vi "Working Point 3 Selection Dialog.vi"(7 "DisplayFilter":u8(ring)=7 items=["K_CHAN_R", "K_CHAN_W", "K_CHAN_RW", "K_CHAN_VOLT", "K_CHAN_FAULT", "K_ALL", "K_CUSTOM", "K_CHAN_R_VIS", "K_CHAN_W_VIS", "K_CHAN_RW_VIS", "K_CHAN_VOLT_VIS", "K_CHAN_FAULT_VIS"], 8 "error in (no error)":errorcluster, 9 "NIVS.System Definition Root":refnum<k24>, 10 "NodePaths":string[](array[string])) -> (0 "error out":errorcluster, 2 "Selected NodePaths":string[](array[string]))   [LabVIEW 2011]
doc: "Use this template to create a dialog box with event handling."
uses:
  NationalInstruments.VeriStand.SystemStorageUI
  NationalInstruments.VeriStand.SystemStorage
  <vilib>/NI Veristand/UI Controls/Single Node Browser/Net Event Data.ctl
  <vilib>/NI Veristand/UI Controls/Single Node Browser/Net Event.ctl
  <vilib>/NI Veristand/UI Controls/Single Node Browser/NI_VS UI Single Node Browser.lvlib
panel:
  in  "Z Value":refnum<k24>(container)
  in  "Y Index":refnum<k24>(container)
  in  "Cancel":bool
  in  "Ok":bool
  in  "X Index":refnum<k24>(container)
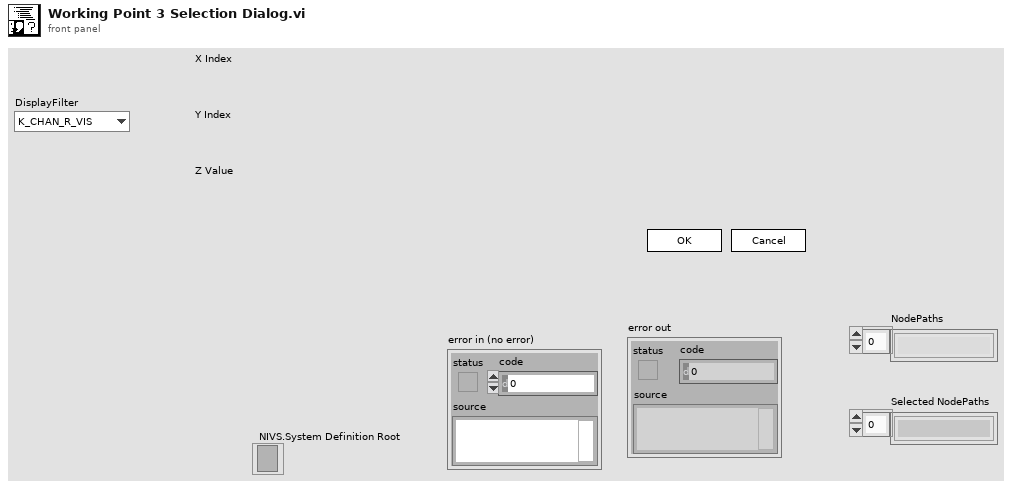
[diagram p1: front panel]
types:
  T1 = typedef "NI_VS UI Single Node Browser.lvlib/Callback Type.ctl" = cluster{"Net Callbacks":refnum<k27>[], "Event":refnum<user-event>}
  T2 = typedef "NI_VS UI Single Node Browser.lvlib/Node Ref.ctl" = refnum<k24>
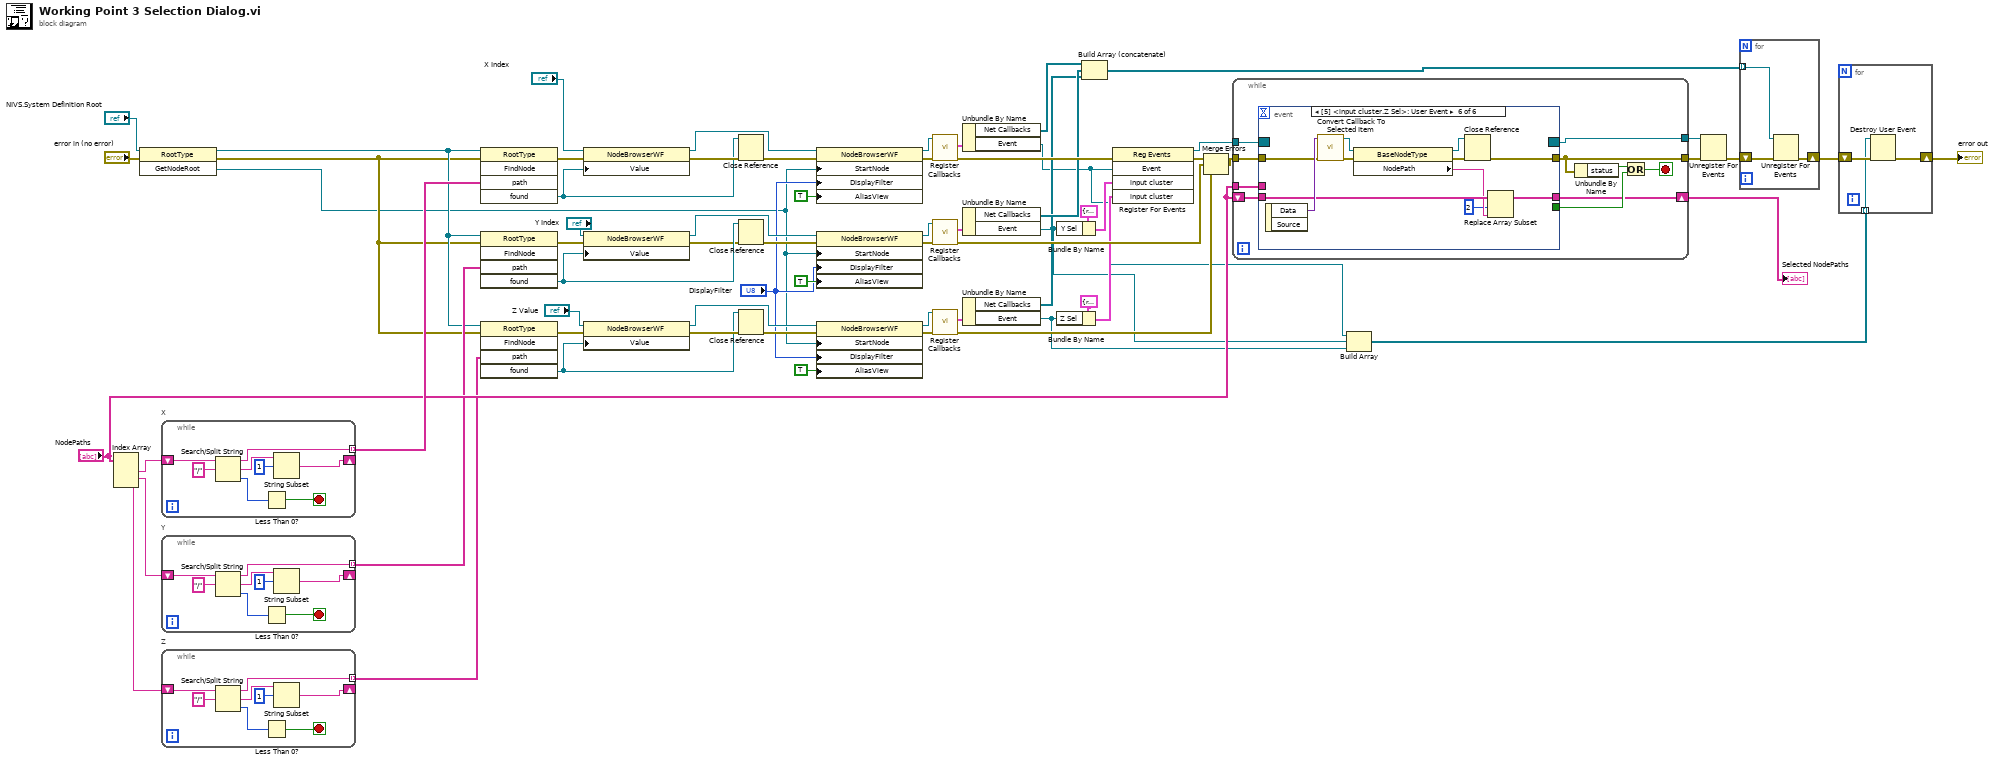
[diagram p0: block diagram]
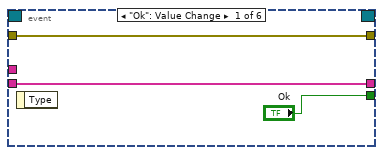
[diagram p2: hidden frame]
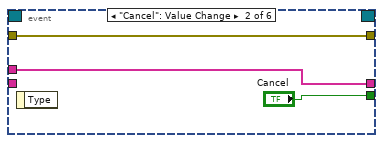
[diagram p3: hidden frame]
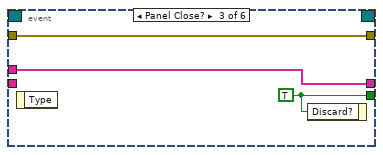
[diagram p4: hidden frame]
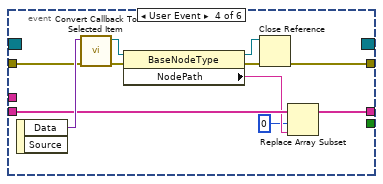
[diagram p5: hidden frame]
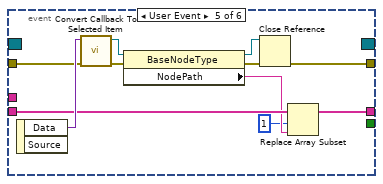
[diagram p6: hidden frame]
diagram:
  n1 = Index Array(array="NodePaths") -> (element #1=w47:string, element #2=w46:string, element #3=w26:string)  [unwired: 3 in]
  n2 = invoke class="RootType" method="GetNodeRoot"(reference="NIVS.System Definition Root", error in="error in (no error)") -> (reference out=w14:refnum<k24>, error out=w13:errorcluster, "GetNodeRoot"=w1:refnum<k24>)  [unwired: 1 in]
  n3 = while "X" {
    tunnel: [w71] -> w53 mode=indexing
    shift-right: [w69] -> _
    shift-left: w47 -> [w75]
    stop <- w72 stop-if-true
    n4 = Search/Split String(string=w75, search string/char (-)="/") -> (substring before match=w71:string, match + rest of string=w70:string, offset of match=w73:i32)  [unwired: 1 in]
    n5 = Less Than 0?(x=w73) -> (x < 0?=w72:bool)
    n6 = String Subset(string=w70, offset (0)=1) -> (substring=w69:string)  [unwired: 1 in]
  }
  n7 = while "Y" {
    tunnel: [w79] -> w34 mode=indexing
    shift-right: [w77] -> _
    shift-left: w46 -> [w83]
    stop <- w80 stop-if-true
    n8 = Search/Split String(string=w83, search string/char (-)="/") -> (substring before match=w79:string, match + rest of string=w78:string, offset of match=w81:i32)  [unwired: 1 in]
    n9 = Less Than 0?(x=w81) -> (x < 0?=w80:bool)
    n10 = String Subset(string=w78, offset (0)=1) -> (substring=w77:string)  [unwired: 1 in]
  }
  n11 = while "Z" {
    tunnel: [w87] -> w12 mode=indexing
    shift-right: [w85] -> _
    shift-left: w26 -> [w91]
    stop <- w88 stop-if-true
    n12 = Search/Split String(string=w91, search string/char (-)="/") -> (substring before match=w87:string, match + rest of string=w86:string, offset of match=w89:i32)  [unwired: 1 in]
    n13 = Less Than 0?(x=w89) -> (x < 0?=w88:bool)
    n14 = String Subset(string=w86, offset (0)=1) -> (substring=w85:string)  [unwired: 1 in]
  }
  n15 = invoke class="RootType" method="FindNode"(reference=w14, error in=w13, "path"=w53) -> (error out=w59:errorcluster, "found"=w54:refnum<k24>)  [unwired: 2 in, 3 out]
  n16 = invoke class="RootType" method="FindNode"(reference=w14, error in=w13, "path"=w34) -> (error out=w40:errorcluster, "found"=w43:refnum<k24>)  [unwired: 2 in, 3 out]
  n17 = invoke class="RootType" method="FindNode"(reference=w14, error in=w13, "path"=w12) -> (error out=w21:errorcluster, "found"=w18:refnum<k24>)  [unwired: 2 in, 3 out]
  n18 = property class="NodeBrowserWF"(reference="X Index", error in=w59, "Value"=w54) -> (reference out=w48:refnum<k24>, error out=w56:errorcluster)
  n19 = property class="NodeBrowserWF"(reference="Y Index", error in=w40, "Value"=w43) -> (reference out=w44:refnum<k24>, error out=w41:errorcluster)
  n20 = property class="NodeBrowserWF"(reference="Z Value", error in=w21, "Value"=w18) -> (reference out=w17:refnum<k24>, error out=w20:errorcluster)
  n21 = Close Reference(reference=w54, error in (no error)=w56) -> (error out=w55:errorcluster)
  n22 = Close Reference(reference=w43, error in (no error)=w41) -> (error out=w42:errorcluster)
  n23 = Close Reference(reference=w18, error in (no error)=w20) -> (error out=w19:errorcluster)
  n24 = property class="NodeBrowserWF"(reference=w48, error in=w55, "StartNode"=w1, "DisplayFilter"="DisplayFilter", "AliasView"=TRUE) -> (reference out=w61:refnum<k24>, error out=w62:errorcluster)
  n25 = property class="NodeBrowserWF"(reference=w44, error in=w42, "StartNode"=w1, "DisplayFilter"="DisplayFilter", "AliasView"=TRUE) -> (reference out=w38:refnum<k24>, error out=w37:errorcluster)
  n26 = property class="NodeBrowserWF"(reference=w17, error in=w19, "StartNode"=w1, "DisplayFilter"="DisplayFilter", "AliasView"=TRUE) -> (reference out=w23:refnum<k24>, error out=w24:errorcluster)
  n27 = call <vilib>:"Register Callbacks.vi"("error in (no error)"=w62, "Single Node Browser"=w61) -> ("error out"=w67:errorcluster, "Callbacks"=w63:T1)  [unwired: 7 in, 1 out]
  n28 = call <vilib>:"Register Callbacks.vi"("error in (no error)"=w37, "Single Node Browser"=w38) -> ("error out"=w30:errorcluster, "Callbacks"=w36:T1)  [unwired: 7 in, 1 out]
  n29 = call <vilib>:"Register Callbacks.vi"("error in (no error)"=w24, "Single Node Browser"=w23) -> ("error out"=w8:errorcluster, "Callbacks"=w25:T1)  [unwired: 7 in, 1 out]
  n30 = Unbundle By Name(w63) -> ("Net Callbacks"=w49:refnum<k27>[], "Event"=w5:refnum<user-event>)
  n31 = Unbundle By Name(w36) -> ("Net Callbacks"=w32:refnum<k27>[], "Event"=w4:refnum<user-event>)
  n32 = Unbundle By Name(w25) -> ("Net Callbacks"=w9:refnum<k27>[], "Event"=w3:refnum<user-event>)
  n33 = Bundle By Name(cluster=cluster{"Y Sel":refnum<user-event>} {"Y Sel"=refnum} ("input cluster"), "Y Sel"=w4) -> (w27:cluster{"Y Sel":refnum<user-event>})
  n34 = Bundle By Name(cluster=cluster{"Z Sel":refnum<user-event>} {"Z Sel"=refnum} ("input cluster"), "Z Sel"=w3) -> (w10:cluster{"Z Sel":refnum<user-event>})
  n35 = Build Array (concatenate)(w49, w32, w9) -> (w33:refnum<k27>[])
  n36 = register-events(error in=w67, w5, w27, w10) -> (reference out=w66:refnum<event-registration>, error out=w57:errorcluster)  [unwired: 1 in]
  n37 = Merge Errors(w57, w30, w8) -> (w31:errorcluster)
  n38 = while {
    tunnel: [w99] -> w52
    tunnel: w31 -> [w100]
    tunnel: w66 -> [w96]
    shift-right: [w95] -> w29
    shift-left: "NodePaths" -> [w94]
    tunnel: "NodePaths" -> [w93]
    tunnel: [w92] -> w51
    stop <- w98 stop-if-true
    n39 = event shown="[5] <input cluster.Z Sel>: User Event" {
      selector: w96 -> [_ _ _ _ _ _]
      dyn-events: [_ _ _ _ _ _] -> w92
      timeout: _ -> [_ _ _ _ _ _]
      tunnel: ["Ok" "Cancel" w110 _ _ _] -> w101
      tunnel: [w104 w106 w109 w119 w130 w141] -> w99
      tunnel: w100 -> [w104 w106 w109 w120 w131 w142]
      tunnel: [w102 w105 w108 w113 w124 w135] -> w95
      tunnel: w94 -> [w102 _ _ w114 w125 w136]
      tunnel: w93 -> [_ w105 w108 _ _ _]
      event "Ok": Value Change {
        n40 = event-data() -> ()  [unwired: 1 in, 1 out]
      }
      event "Cancel": Value Change {
        n41 = event-data() -> ()  [unwired: 1 in, 1 out]
      }
      event Panel Close? {
        w110 = TRUE ("Cancel")
        n42 = event-data() -> ()  [unwired: 1 in, 1 out]
        n43 = event-data("Discard?"=w110) -> ()  [unwired: 1 in, 1 out]
      }
      event User Event {
        n44 = event-data() -> ("Data"=w121:variant)  [unwired: 1 in, 1 out]
        n45 = call <vilib>:"Convert Callback To Selected Item.vi"("error in"=w120, "Data"=w121) -> ("error out"=w115:errorcluster, "Selected Item"=w118:T2)  [unwired: 8 in]
        n46 = property class="BaseNodeType"(reference=w118, error in=w115) -> (reference out=w117:T2, error out=w116:errorcluster, "NodePath"=w112:string)
        n47 = Close Reference(reference=w117, error in (no error)=w116) -> (error out=w119:errorcluster)
        n48 = Replace Array Subset(array=w114, new element=w112, index=0) -> (w113:string[])
      }
      event User Event {
        n49 = event-data() -> ("Data"=w132:variant)  [unwired: 1 in, 1 out]
        n50 = call <vilib>:"Convert Callback To Selected Item.vi"("error in"=w131, "Data"=w132) -> ("error out"=w126:errorcluster, "Selected Item"=w129:T2)  [unwired: 8 in]
        n51 = property class="BaseNodeType"(reference=w129, error in=w126) -> (reference out=w128:T2, error out=w127:errorcluster, "NodePath"=w123:string)
        n52 = Close Reference(reference=w128, error in (no error)=w127) -> (error out=w130:errorcluster)
        n53 = Replace Array Subset(array=w125, new element=w123, index=1) -> (w124:string[])
      }
      event User Event {
        n54 = event-data() -> ("Data"=w143:variant)  [unwired: 1 in, 1 out]
        n55 = call <vilib>:"Convert Callback To Selected Item.vi"("error in"=w142, "Data"=w143) -> ("error out"=w137:errorcluster, "Selected Item"=w140:T2)  [unwired: 8 in]
        n56 = property class="BaseNodeType"(reference=w140, error in=w137) -> (reference out=w139:T2, error out=w138:errorcluster, "NodePath"=w134:string)
        n57 = Close Reference(reference=w139, error in (no error)=w138) -> (error out=w141:errorcluster)
        n58 = Replace Array Subset(array=w136, new element=w134, index=2) -> (w135:string[])
      }
    }
    n59 = Unbundle By Name(w99) -> ("status"=w97:bool)
    n60 = Or(x=w97, y=w101) -> (x .or. y?=w98:bool)
  }
  "Selected NodePaths" <- w29
  n61 = Build Array(w5, w4, w3) -> (w2:refnum<user-event>[])
  n62 = Unregister For Events(event registration refnum=w51, error in=w52) -> (error out=w50:errorcluster)
  n63 = for {
    tunnel: w33 -> [w145] mode=indexing
    shift-right: [w144] -> w7
    shift-left: w50 -> [w146]
    n64 = Unregister For Events(event registration refnum=w145, error in=w146) -> (error out=w144:errorcluster)
  }
  n65 = for {
    shift-right: [w148] -> w6
    shift-left: w7 -> [w149]
    tunnel: w2 -> [w147] mode=indexing
    n66 = Destroy User Event(user event=w147, error in=w149) -> (error out=w148:errorcluster)
  }
  "error out" <- w6
